vi "参数设置页.vi"() -> ()   [LabVIEW 2016, in "斯坦道氨氮V2.lvlib"]
uses:
  <vilib>/Plasmionique/MB Master/MB_Master/MB_Master.lvclass
  <vilib>/ptbypt/NI_PtbyPt.lvlib
panel:
  out "连接状态":bool
  out "低量程上限":dbl caption="低量程上限："
  out "数据刷新时间":string
  in  "通讯连接":bool=TRUE
  out "MB table":enum32{"Serial", "TCP"}(tab)
  in  "请选择串口:":refnum<visa-resource-name>
  in  "IP":string="127.0.0.1"
  in  "PORT":string="1001"
  in  "通信方式选择":enum16{"串口", "TCP"}(ring)
  in  "刷新":bool
  in  "测量模式":enum16{"跨度核查", "水样测量", "零点核查", "标样核查", "加标回收"}(ring)
  in  "参数下拉列表":u16(ring)
  in  "量程下拉列表":enum16{"低量程", "高量程"}(ring)
  in  "测试流程路径":path=path "data/流程.xml"
  in  "标样核查量程模式":T1 caption="标样核查："
  in  "加标回收量程模式":T1 caption="加标回收："
  in  "跨度核查量程模式":T1 caption="跨度核查："
  in  "零点核查量程模式":T1 caption="零点核查："
  in  "水样测试量程模式":T1 caption="水样测试："
  out "阈值（高->低）":dbl caption="阈值（高->低）："
  out "阈值（低->高）":dbl caption="阈值（低->高）："
  out "量程下限":dbl caption="量程下限："
  out "高量程上限":dbl caption="高量程上限："
  out "检出限":dbl caption="检出限："
  out "曲线截距":dbl caption="曲线截距：" format="%#.6f"
  out "曲线斜率":dbl caption="曲线斜率：" format="%#.6f"
  out "二次多项式系数":dbl caption="二次多项式系数：" format="%#.6f"
  out "消解时长":dbl caption="消解时长："
  out "消解温度":dbl caption="消解温度："
  out "测量精度":u16 caption="测量精度："
  in  "标样核查标液浓度":dbl caption="标样核查标液浓度："
  in  "跨度核查标液浓度":dbl caption="跨度核查标液浓度："
  in  "零点核查标液浓度":dbl caption="零点核查标液浓度："
  in  "跨度值":dbl caption="跨度值："
  # "自动量程设置"
  # "mg/L"
  # "mg/L"
  # "mg/L"
  # "mg/L"
  # "mg/L"
  # "mg/L"
  # "min"
  # "℃"
  # "mg/L"
  # "mg/L"
  # "mg/L"
  # "mg/L"
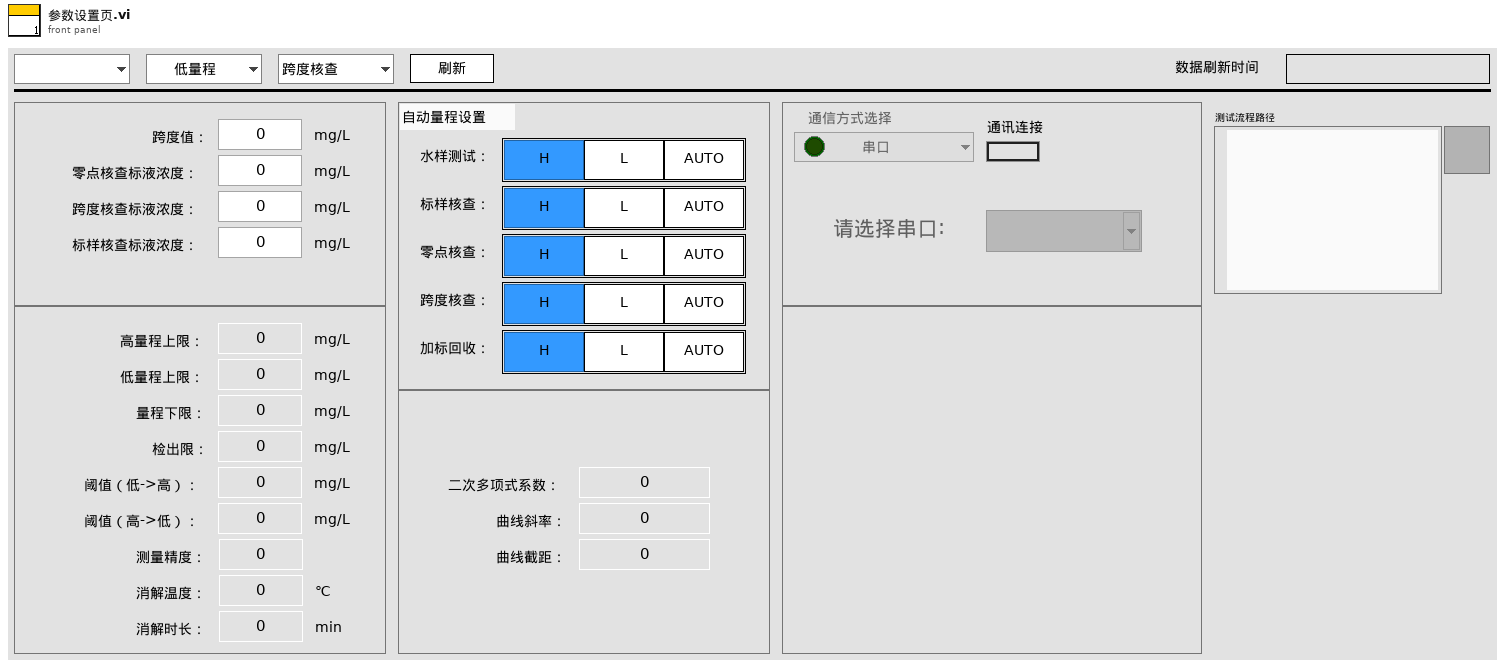
[diagram p1: front panel]
types:
  T1 = typedef "斯坦道氨氮V2.lvlib/量程设置.ctl" = enum32{"H", "L", "AUTO"}
  T2 = enum16{"跨度核查", "水样测量", "零点核查", "标样核查", "加标回收", "快捷测试", "空白校准", "标样校准"}
  T3 = typedef "LVStringsAndValuesArrayTypeDef_U16.ctl" = cluster{"String":string, "Value":u16}[]
  T4 = enum8{"Enabled", "Disabled", "Disabled and Grayed Out"}
  T5 = cluster{"总磷跨度值":dbl, "总磷零点标准液浓度":dbl, "总磷跨度标准液浓度":dbl, "总磷标准液标准浓度":dbl, "总氮跨度值":dbl, "总氮零点标准液浓度":dbl, "总氮跨度标准液浓度":dbl, "总氮标准液标准浓度":dbl, "氨氮跨度值":dbl, "氨氮零点标准液浓度":dbl, "氨氮跨度标准液浓度":dbl, "氨氮标准液标准浓度":dbl}
  T6 = cluster{"水样测试量程模式":enum16{"H", "L", "AUTO"}, "空白核查量程模式":enum16{"H", "L", "AUTO"}, "跨度核查量程模式":enum16{"H", "L", "AUTO"}, "加标回收量程模式":enum16{"H", "L", "AUTO"}, "标样核查量程模式":enum16{"H", "L", "AUTO"}}
  T7 = cluster{"水样测试量程模式":u16, "空白核查量程模式":u16, "跨度核查量程模式":u16, "加标回收量程模式":u16, "标样核查量程模式":u16}
  T8 = cluster{"精度":dbl, "检出限":dbl, "量程上限":dbl, "量程下限":dbl}
  T9 = cluster{"水样测试量程模式":T1, "零点核查量程模式":T1, "跨度核查量程模式":T1, "加标回收量程模式":T1, "标样核查量程模式":T1}
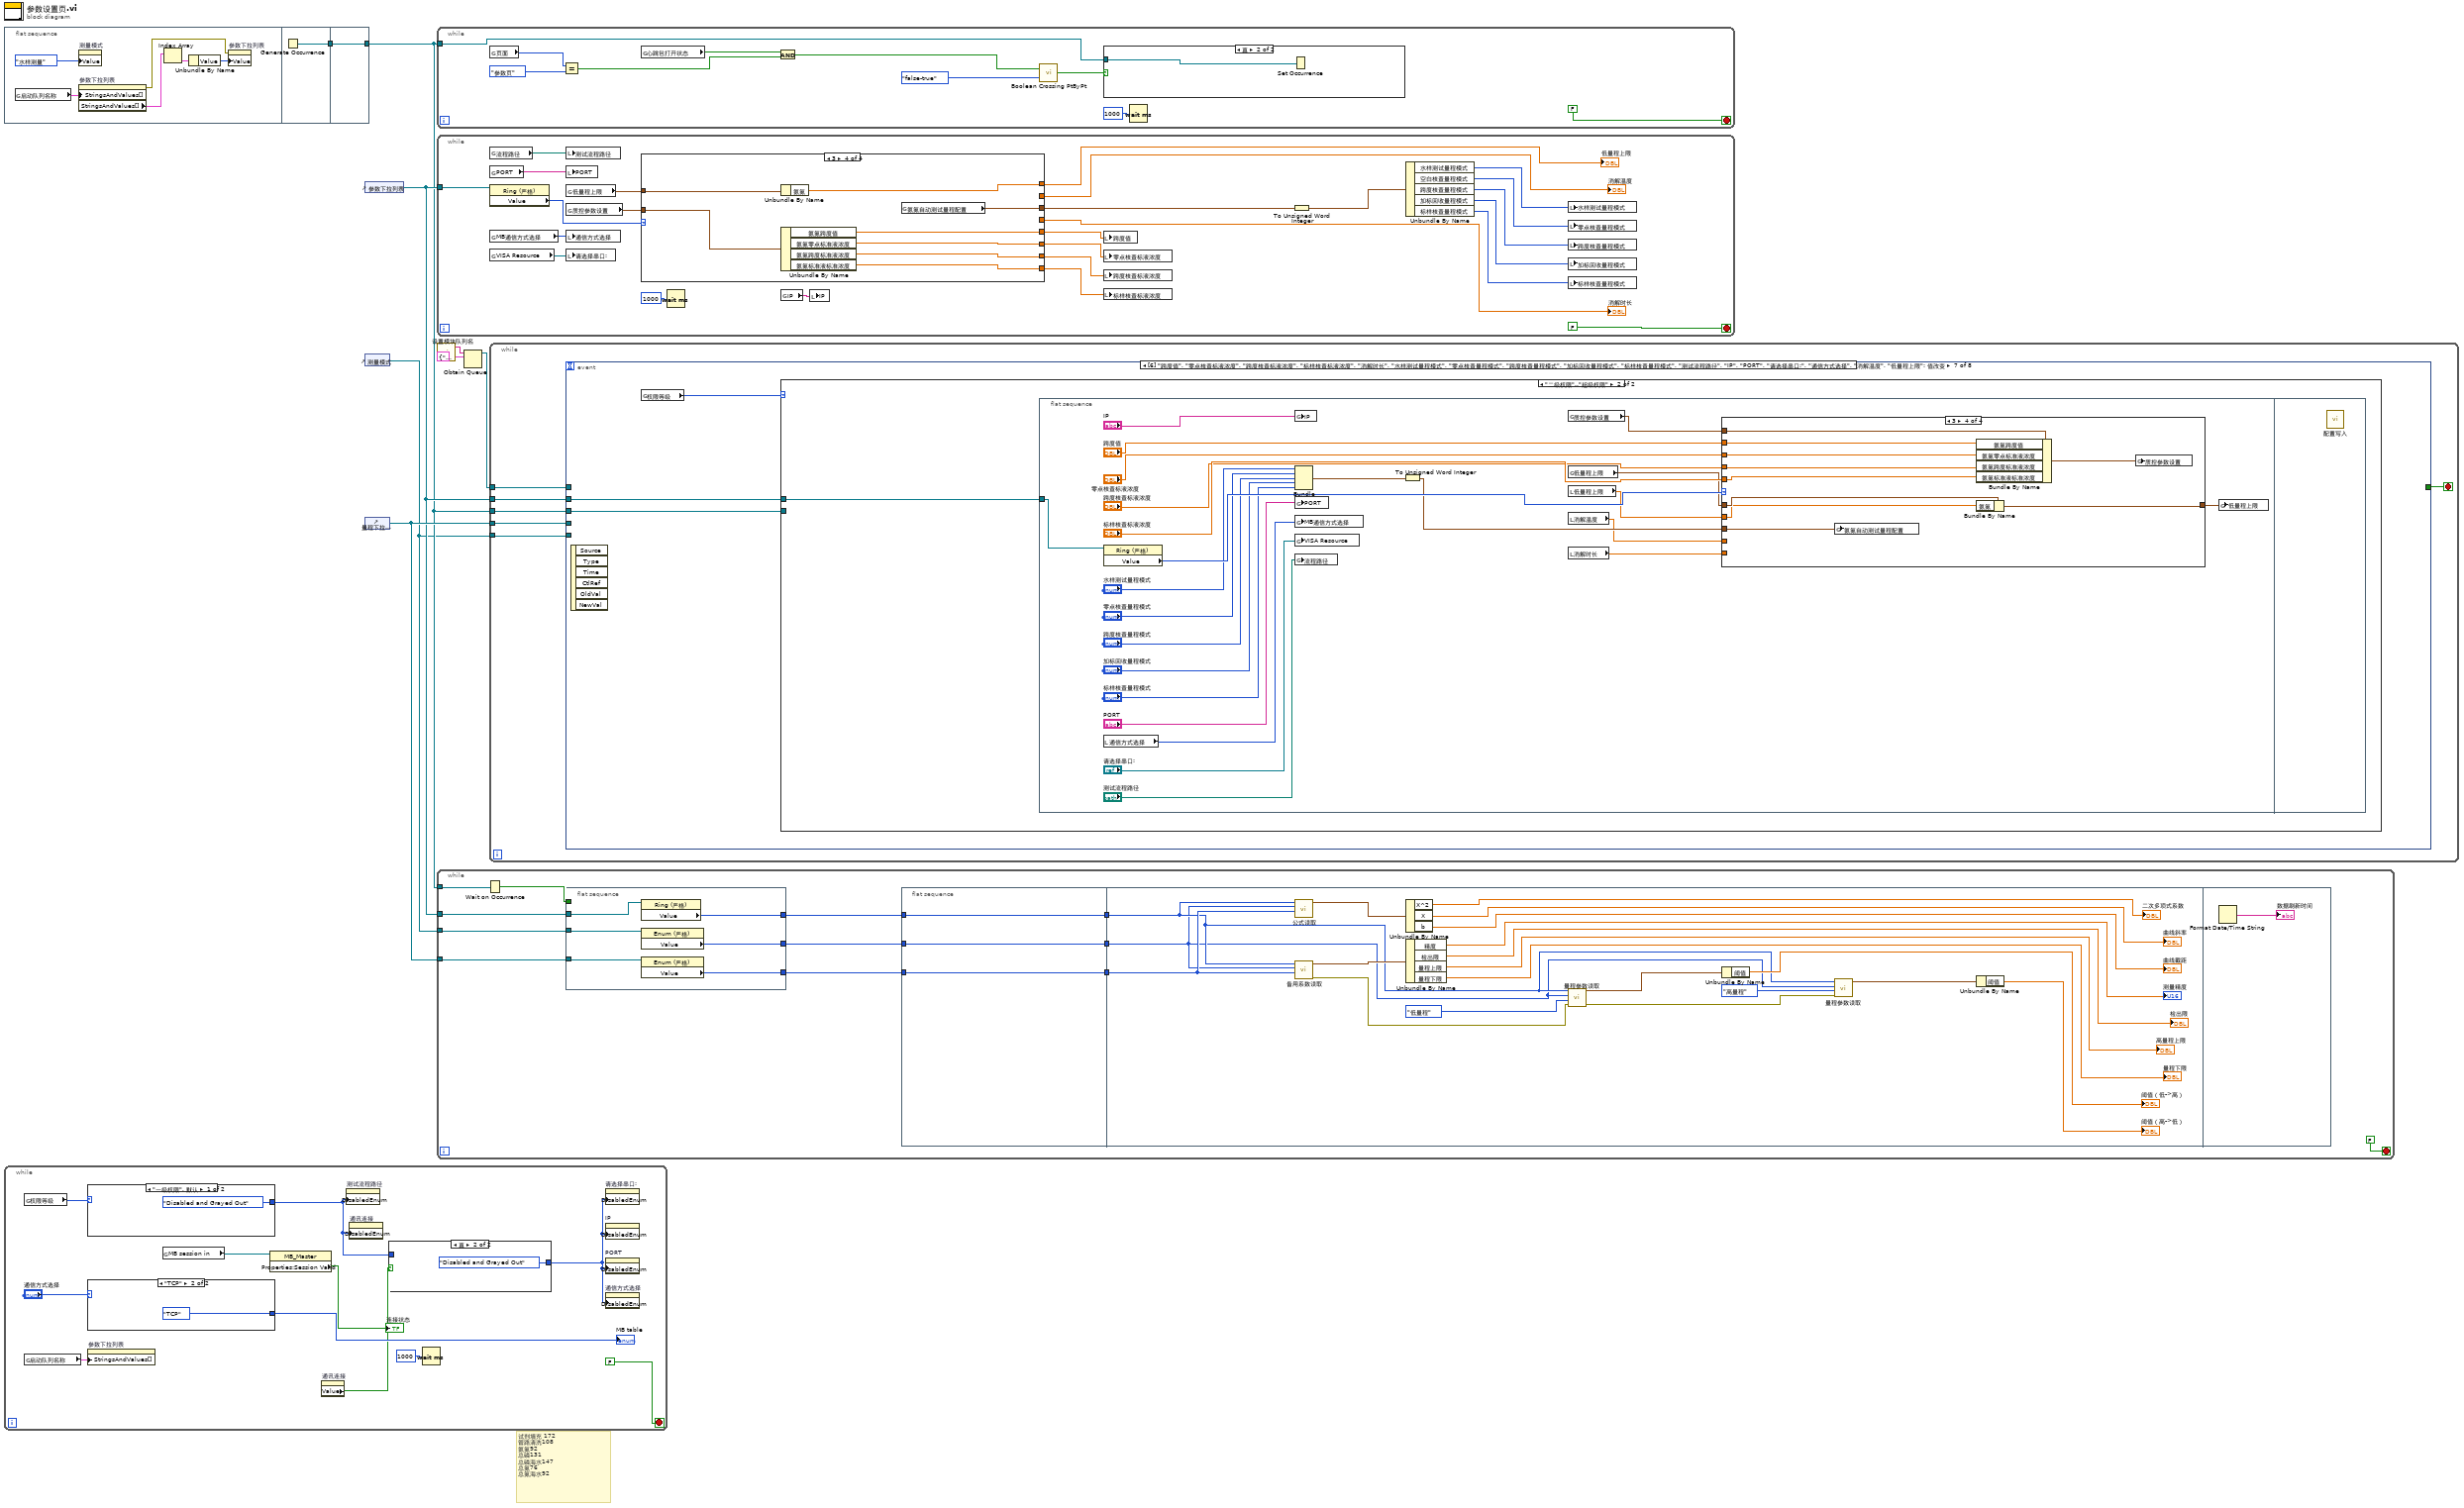
[diagram p0: block diagram]
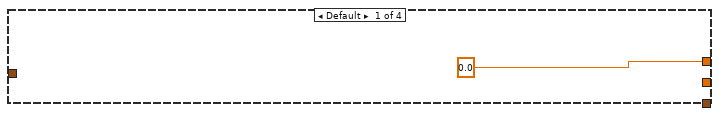
[diagram p3: hidden frame]
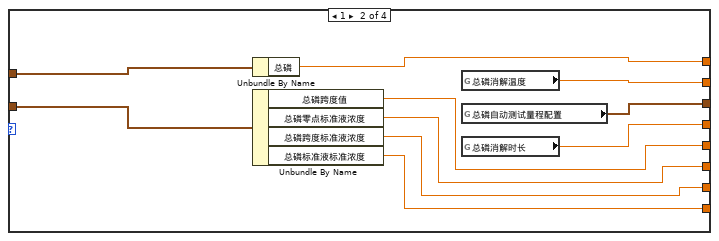
[diagram p4: hidden frame]
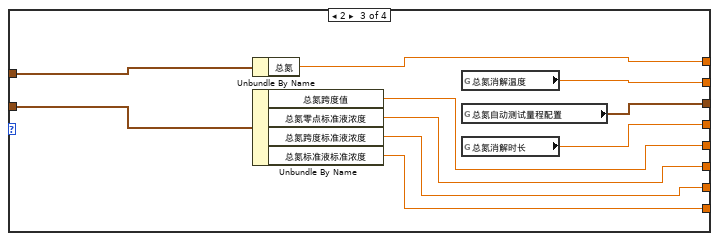
[diagram p5: hidden frame]
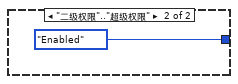
[diagram p6: hidden frame]
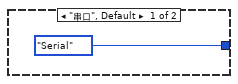
[diagram p7: hidden frame]
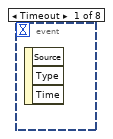
[diagram p9: hidden frame]
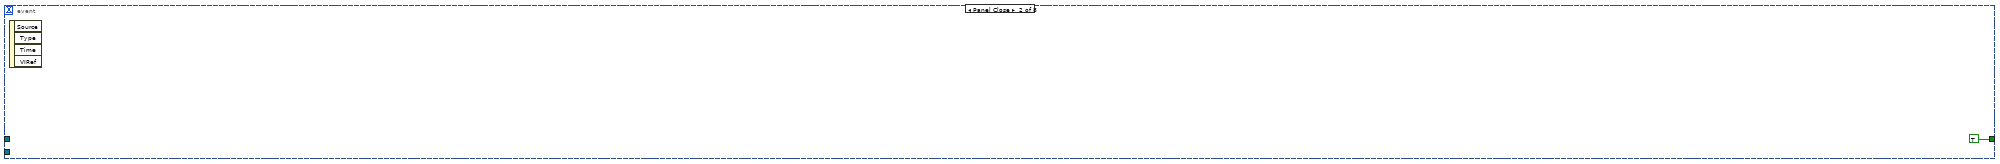
[diagram p10: hidden frame]
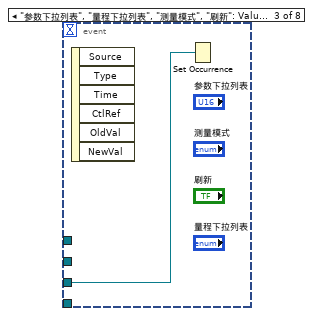
[diagram p11: hidden frame]
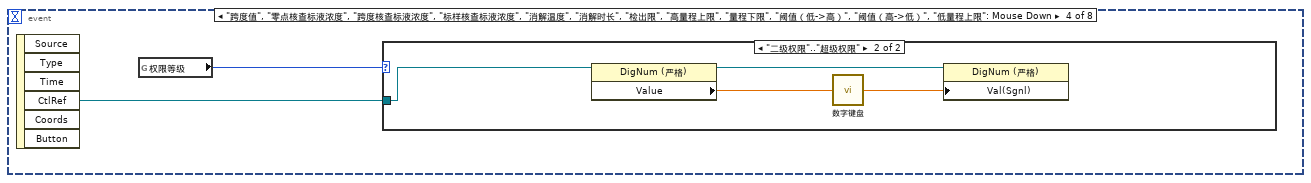
[diagram p12: hidden frame]
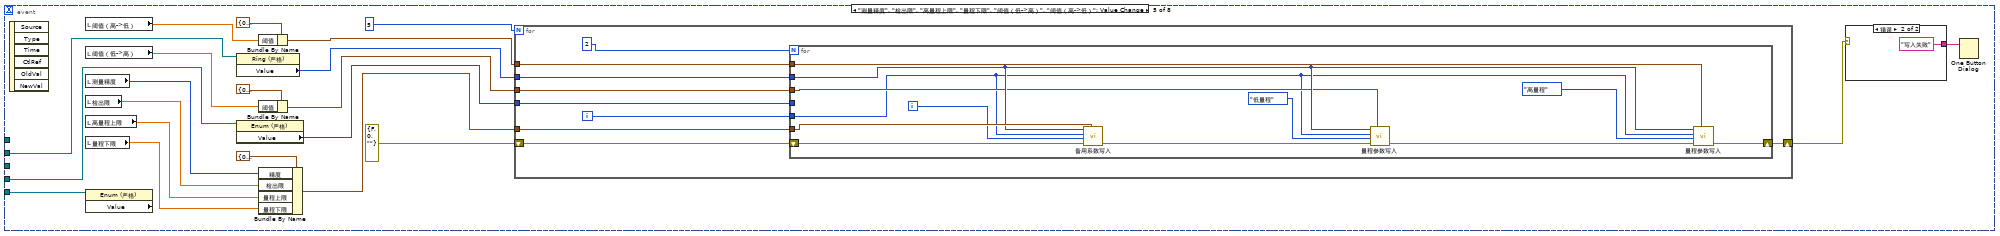
[diagram p14: hidden frame]
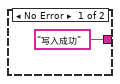
[diagram p15: hidden frame]
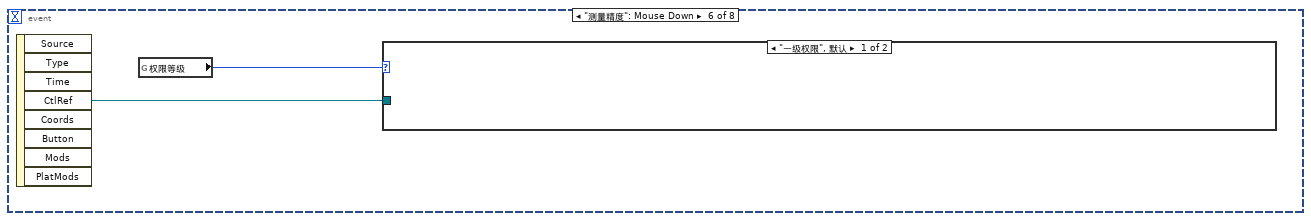
[diagram p16: hidden frame]
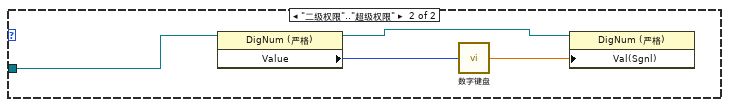
[diagram p17: hidden frame]
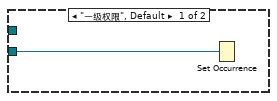
[diagram p18: hidden frame]
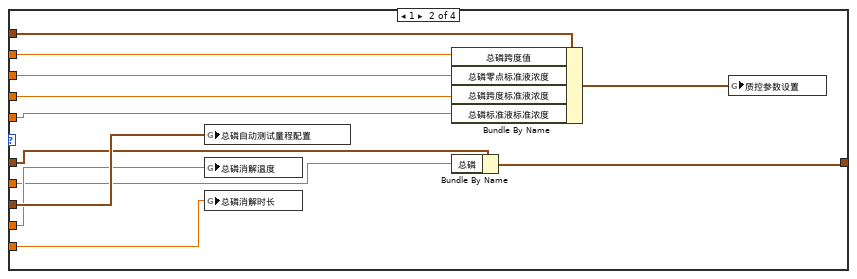
[diagram p20: hidden frame]
diagram:
  # "试剂填充 172 \n管路清洗108\n氨氮92\n总磷131\n总磷海水147\n总氮76\n总氮海水92"
  n1 = flat-sequence {
    tunnel: [w15] -> w8
    tunnel: [w16] -> w2
    tunnel: w8 -> [w16]
    frame #0 {
      n2 = global read "总磷总氮断电保存全局变量.vi" "启动队列名称"() -> (w10:cluster{"String":string, "Value":u16}[])
      n3 = property on="测量模式" class="Enum (严格)"("Value"=T2."水样测量" ("测量模式")) -> ()  [unwired: 2 in, 2 out]
      n4 = property on="参数下拉列表" class="Ring (严格)"("StringsAndValues[]"=w10) -> (error out=w13:errorcluster, "StringsAndValues[]"=w11:T3)  [unwired: 2 in, 1 out]
      n5 = Index Array(array=w11) -> (element=w12:cluster{"String":string, "Value":u16})  [unwired: 1 in]
      n6 = Unbundle By Name(w12) -> ("Value"=w14:u16)
      n7 = property on="参数下拉列表" class="Ring (严格)"(error in=w13, "Value"=w14) -> ()  [unwired: 1 in, 2 out]
    }
    frame #1 {
      n8 = Generate Occurrence() -> (w15:refnum<k4>)
    }
    frame #2 {
    }
  }
  n9 = while {
    stop <- FALSE stop-if-true
    n10 = global read "VAR总磷总氮全局变量.vi" "权限等级"() -> (w21:enum16{"一级权限", "二级权限", "三级权限", "超级权限"})
    n11 = global read "总磷总氮断电保存全局变量.vi" "启动队列名称"() -> (w19:cluster{"String":string, "Value":u16}[])
    n12 = case shown="\"一级权限\", 默认" w21 {
      tunnel: [T4."Disabled and Grayed Out" ("禁用") T4."Enabled" ("禁用")] -> w20
      frame "一级权限", Default {
      }
      frame "二级权限".."超级权限" {
      }
    }
    n13 = case shown="\"TCP\"" "通信方式选择" {
      tunnel: [enum32{"Serial", "TCP"}."Serial" ("MB table") enum32{"Serial", "TCP"}."TCP" ("MB table")] -> w23
      frame "串口", Default {
      }
      frame "TCP" {
      }
    }
    "MB table" <- w23
    n14 = property on="参数下拉列表" class="Ring (严格)"("StringsAndValues[]"=w19) -> ()  [unwired: 2 in, 2 out]
    n15 = global read "VAR总磷总氮全局变量.vi" "MB session in"() -> (w26:refnum<class "MB_Master.lvclass">)
    n16 = property class="MB_Master"(reference=w26) -> ("Properties:Session Valid"=→"连接状态":bool)  [unwired: 1 in, 2 out]
    n17 = property on="通讯连接" class="Bool (严格)"() -> ("Value"=w17:bool)  [unwired: 2 in, 2 out]
    n18 = property on="测试流程路径" class="Path"("DisabledEnum"=w20) -> ()  [unwired: 2 in, 2 out]
    n19 = property on="通讯连接" class="Bool (严格)"("DisabledEnum"=w20) -> ()  [unwired: 2 in, 2 out]
    n20 = case shown="真" w17 {
      tunnel: [w32 T4."Disabled and Grayed Out" ("禁用")] -> w24
      tunnel: w20 -> [w32 _]
      frame False {
      }
      frame True {
      }
    }
    n21 = Wait (ms)(milliseconds to wait=u32 1000 ("等待时间（毫秒）")) -> ()  [unwired: 1 out]
    n22 = property on="请选择串口:" class="VISAName"("DisabledEnum"=w24) -> ()  [unwired: 2 in, 2 out]
    n23 = property on="IP" class="Str"("DisabledEnum"=w24) -> ()  [unwired: 2 in, 2 out]
    n24 = property on="PORT" class="Str"("DisabledEnum"=w24) -> ()  [unwired: 2 in, 2 out]
    n25 = property on="通信方式选择" class="Enum (严格)"("DisabledEnum"=w24) -> ()  [unwired: 2 in, 2 out]
  }
  n26 = control-ref of="参数下拉列表"() -> (w3:refnum<vi>)
  n27 = control-ref of="测量模式"() -> (w1:refnum<vi>)
  n28 = control-ref of="量程下拉列表"() -> (w4:refnum<vi>)
  n29 = while {
    tunnel: w2 -> [w40]
    stop <- FALSE stop-if-true
    n30 = global read "VAR总磷总氮全局变量.vi" "页面"() -> (w42:enum16{"主页", "参数页", "校准页"})
    n31 = Equal?(x=w42, y=enum16{"主页", "参数页", "校准页"}."参数页" ("页面")) -> (x = y?=w41:bool)
    n32 = global read "VAR总磷总氮全局变量.vi" "心跳包打开状态"() -> (w36:bool)
    n33 = And(x=w36, y=w41) -> (x .and. y?=w37:bool)
    n34 = call <vilib>:"Boolean Crossing PtByPt.vi"("direction"=enum16{"either", "false-true", "true-false"}."false-true", "input"=w37) -> ("crossing"=w35:bool)  [unwired: 1 in]
    n35 = case shown="真" w35 {
      tunnel: w40 -> [_ w44]
      frame False {
      }
      frame True {
        n36 = Set Occurrence(w44) -> ()
      }
    }
    n37 = Wait (ms)(milliseconds to wait=u32 1000 ("等待时间（毫秒）")) -> ()  [unwired: 1 out]
  }
  n38 = while {
    tunnel: w3 -> [w49]
    stop <- FALSE stop-if-true
    n39 = global read "总磷总氮断电保存全局变量.vi" "流程路径"() -> (w64:path)
    n40 = global read "总磷总氮断电保存全局变量.vi" "PORT"() -> (w66:string)
    n41 = property class="Ring (严格)"(reference=w49) -> ("Value"=w48:u16)  [unwired: 1 in, 2 out]
    n42 = global read "总磷总氮断电保存全局变量.vi" "MB通信方式选择"() -> (w63:enum16{"串口", "TCP"})
    n43 = global read "总磷总氮断电保存全局变量.vi" "VISA Resource"() -> (w67:refnum<visa-resource-name>)
    n44 = local write "测试流程路径"(w64) -> ()
    n45 = local write "PORT"(w66) -> ()
    n46 = global read "总磷总氮断电保存全局变量.vi" "低量程上限"() -> (w46:cluster{"总磷":dbl, "总氮":dbl, "氨氮":dbl})
    n47 = global read "总磷总氮断电保存全局变量.vi" "质控参数设置"() -> (w58:T5)
    n48 = local write "通信方式选择"(w63) -> ()
    n49 = local write "请选择串口:"(w67) -> ()
    n50 = case shown="3" w48 {
      tunnel: [_ w80 w90 w98] -> w56
      tunnel: [_ w79 w89 _] -> w57
      tunnel: w58 -> [_ w78 w88 w97]
      tunnel: [_ w77 w87 w96] -> w59
      tunnel: [_ w76 w86 w95] -> w60
      tunnel: [_ w75 w85 w94] -> w61
      tunnel: [_ w74 w84 w93] -> w62
      tunnel: [_ w73 w83 _] -> w47
      tunnel: w46 -> [_ w72 w82 w92]
      tunnel: [0.0 ("COD") w71 w81 w91] -> w45
      frame Default {
      }
      frame 1 {
        n51 = Unbundle By Name(w72) -> ("总磷"=w71:dbl)
        n52 = Unbundle By Name(w78) -> ("总磷跨度值"=w77:dbl, "总磷零点标准液浓度"=w76:dbl, "总磷跨度标准液浓度"=w75:dbl, "总磷标准液标准浓度"=w74:dbl)
        n53 = global read "总磷总氮断电保存全局变量.vi" "总磷消解温度"() -> (w73:dbl)
        n54 = global read "总磷总氮断电保存全局变量.vi" "总磷自动测试量程配置"() -> (w80:T6)
        n55 = global read "总磷总氮断电保存全局变量.vi" "总磷消解时长"() -> (w79:dbl)
      }
      frame 2 {
        n56 = Unbundle By Name(w82) -> ("总氮"=w81:dbl)
        n57 = Unbundle By Name(w88) -> ("总氮跨度值"=w87:dbl, "总氮零点标准液浓度"=w86:dbl, "总氮跨度标准液浓度"=w85:dbl, "总氮标准液标准浓度"=w84:dbl)
        n58 = global read "总磷总氮断电保存全局变量.vi" "总氮消解温度"() -> (w83:dbl)
        n59 = global read "总磷总氮断电保存全局变量.vi" "总氮自动测试量程配置"() -> (w90:T6)
        n60 = global read "总磷总氮断电保存全局变量.vi" "总氮消解时长"() -> (w89:dbl)
      }
      frame 3 {
        n61 = Unbundle By Name(w92) -> ("氨氮"=w91:dbl)
        n62 = Unbundle By Name(w97) -> ("氨氮跨度值"=w96:dbl, "氨氮零点标准液浓度"=w95:dbl, "氨氮跨度标准液浓度"=w94:dbl, "氨氮标准液标准浓度"=w93:dbl)
        n63 = global read "总磷总氮断电保存全局变量.vi" "氨氮自动测试量程配置"() -> (w98:T6)
      }
    }
    "消解时长" <- w57
    "消解温度" <- w47
    "低量程上限" <- w45
    n64 = Wait (ms)(milliseconds to wait=u32 1000 ("等待时间（毫秒）")) -> ()  [unwired: 1 out]
    n65 = global read "总磷总氮断电保存全局变量.vi" "IP"() -> (w65:string)
    n66 = local write "IP"(w65) -> ()
    n67 = local write "跨度值"(w59) -> ()
    n68 = local write "零点核查标液浓度"(w60) -> ()
    n69 = local write "跨度核查标液浓度"(w61) -> ()
    n70 = local write "标样核查标液浓度"(w62) -> ()
    n71 = To Unsigned Word Integer(number=w56) -> (unsigned 16bit integer=w55:T7)
    n72 = Unbundle By Name(w55) -> ("水样测试量程模式"=w54:u16, "空白核查量程模式"=w52:u16, "跨度核查量程模式"=w51:u16, "加标回收量程模式"=w50:u16, "标样核查量程模式"=w53:u16)
    n73 = local write "水样测试量程模式"(w54) -> ()
    n74 = local write "零点核查量程模式"(w52) -> ()
    n75 = local write "跨度核查量程模式"(w51) -> ()
    n76 = local write "加标回收量程模式"(w50) -> ()
    n77 = local write "标样核查量程模式"(w53) -> ()
  }
  n78 = call "设置模块队列名.vi"() -> ("Msg"=w6:string)  [unwired: 5 in]
  n79 = while {
    tunnel: w3 -> [w109]
    tunnel: w4 -> [w108]
    tunnel: w1 -> [w107]
    tunnel: w2 -> [w106]
    stop <- FALSE stop-if-true
    n80 = Wait on Occurrence(2:w106) -> (0:w100:bool)  [unwired: 2 in]
    n81 = flat-sequence {
      tunnel: w109 -> [w116]
      tunnel: w108 -> [w115]
      tunnel: w107 -> [w114]
      tunnel: [w113] -> w103
      tunnel: [w112] -> w102
      tunnel: [w111] -> w101
      tunnel: w100 -> [_]
      frame #0 {
        n82 = property class="Ring (严格)"(reference=w116) -> ("Value"=w113:u16)  [unwired: 1 in, 2 out]
        n83 = property class="Enum (严格)"(reference=w114) -> ("Value"=w111:enum16{"跨度核查", "水样测量", "零点核查", "标样核查", "加标回收"})  [unwired: 1 in, 2 out]
        n84 = property class="Enum (严格)"(reference=w115) -> ("Value"=w112:enum16{"低量程", "高量程"})  [unwired: 1 in, 2 out]
      }
    }
    n85 = flat-sequence {
      tunnel: [w119] -> w105
      tunnel: [w118] -> w104
      tunnel: w103 -> [w117]
      tunnel: w102 -> [w119]
      tunnel: w101 -> [w118]
      tunnel: [w117] -> w99
      tunnel: w105 -> [w134]
      tunnel: w104 -> [w124]
      tunnel: w99 -> [w125]
      frame #0 {
      }
      frame #1 {
        n86 = call "公式读取.vi"("量程下拉列表"=w134, "测量模式"=w124, "参数下拉列表"=w125) -> ("公式"=w139:cluster{"X^2":dbl, "X":dbl, "b":dbl})  [unwired: 7 in, 1 out]
        n87 = call "备用系数读取.vi"("量程下拉列表"=w134, "测量模式"=w124, "参数下拉列表"=w125) -> ("error out"=w135:errorcluster, "备用系数"=w133:T8)  [unwired: 7 in]
        n88 = Unbundle By Name(w139) -> ("X^2"=→"二次多项式系数":dbl, "X"=→"曲线斜率":dbl, "b"=→"曲线截距":dbl)
        n89 = Unbundle By Name(w133) -> ("精度"=→"测量精度":dbl, "检出限"=→"检出限":dbl, "量程上限"=→"高量程上限":dbl, "量程下限"=→"量程下限":dbl)
        n90 = call "量程参数读取.vi"("error in (no error)"=w135, "量程下拉列表"=enum16{"低量程", "高量程"}."低量程", "测量模式"=w124, "参数下拉列表"=w125) -> ("error out"=w126:errorcluster, "量程切换阈值"=w132:cluster{"阈值":dbl, "标液浓度":dbl})  [unwired: 6 in]
        n91 = Unbundle By Name(w132) -> ("阈值"=→"阈值（低->高）":dbl)
        n92 = call "量程参数读取.vi"("error in (no error)"=w126, "量程下拉列表"=enum16{"低量程", "高量程"}."高量程", "测量模式"=w124, "参数下拉列表"=w125) -> ("量程切换阈值"=w121:cluster{"阈值":dbl, "标液浓度":dbl})  [unwired: 6 in, 1 out]
        n93 = Unbundle By Name(w121) -> ("阈值"=→"阈值（高->低）":dbl)
      }
      frame #2 {
        n94 = Format Date/Time String() -> (date/time string=→"数据刷新时间":string)  [unwired: 3 in]
      }
    }
  }
  n95 = Obtain Queue(name (unnamed)=w6, element data type=cluster{"命令":string, "data":variant} {"命令"="", "data"=variant}) -> (queue out=w5:refnum<queue>)  [unwired: 3 in, 2 out]
  n96 = while {
    tunnel: w2 -> [w145]
    tunnel: w3 -> [w144]
    tunnel: w5 -> [w143]
    tunnel: w4 -> [w142]
    tunnel: w1 -> [w141]
    stop <- w146 stop-if-true
    n97 = event shown="[6] \"跨度值\", \"零点核查标液浓度\", \"跨度核查标液浓度\", \"标样核查标液浓度\", \"消解时长\", \"水样测试量程模式\", \"零点核查量程模式\", \"跨度核查量程模式\", \"加标回收量程模式\", \"标样核查量程模式\", \"测试流程路径\", \"IP\", \"PORT\", \"请选择串口:\", \"通信方式选择\", \"消解温度\", \"低量程上限\": 值改变" {
      selector: _ -> [_ _ _ _ _ _ _ _]
      dyn-events: _ -> [_ _ _ _ _ _ _ _]
      timeout: _ -> [_ _ _ _ _ _ _ _]
      tunnel: [_ TRUE _ _ _ _ _ _] -> w146
      tunnel: w145 -> [_ _ w148 _ _ _ w205 _]
      tunnel: w144 -> [_ _ _ _ w175 _ w207 _]
      tunnel: w143 -> [_ _ _ _ _ _ _ w270]
      tunnel: w142 -> [_ _ _ _ w168 _ _ _]
      tunnel: w141 -> [_ _ _ _ w169 _ _ _]
      event Timeout {
        n98 = event-data() -> ()  [unwired: 1 in, 3 out]
      }
      event Panel Close {
        n99 = event-data() -> ()  [unwired: 1 in, 4 out]
      }
      event "参数下拉列表", "量程下拉列表", "测量模式", "刷新": Value Change {
        n100 = event-data() -> ()  [unwired: 1 in, 6 out]
        n101 = Set Occurrence(w148) -> ()
      }
      event "跨度值", "零点核查标液浓度", "跨度核查标液浓度", "标样核查标液浓度", "消解温度", "消解时长", "检出限", "高量程上限", "量程下限", "阈值（低->高）", "阈值（高->低）", "低量程上限": Mouse Down {
        n102 = event-data() -> ("CtlRef"=w150:refnum<vi>)  [unwired: 1 in, 5 out]
        n103 = global read "VAR总磷总氮全局变量.vi" "权限等级"() -> (w149:enum16{"一级权限", "二级权限", "三级权限", "超级权限"})
        n104 = case shown="\"二级权限\"..\"超级权限\"" w149 {
          tunnel: w150 -> [_ w154]
          frame "一级权限", Default {
          }
          frame "二级权限".."超级权限" {
            n105 = property class="DigNum (严格)"(reference=w154) -> (reference out=w152:refnum<vi>, "Value"=w153:dbl)  [unwired: 1 in, 1 out]
            n106 = call "数字键盘.vi"("OldNumber"=w153) -> ("NewNumber"=w151:dbl)
            n107 = property class="DigNum (严格)"(reference=w152, "Val(Sgnl)"=w151) -> ()  [unwired: 1 in, 2 out]
          }
        }
      }
      event "测量精度", "检出限", "高量程上限", "量程下限", "阈值（低->高）", "阈值（高->低）": Value Change {
        n108 = event-data() -> ()  [unwired: 1 in, 6 out]
        n109 = local read "阈值（高->低）"() -> (w158:dbl)
        n110 = local read "阈值（低->高）"() -> (w163:dbl)
        n111 = local read "测量精度"() -> (w171:u16)
        n112 = local read "检出限"() -> (w172:dbl)
        n113 = local read "高量程上限"() -> (w174:dbl)
        n114 = local read "量程下限"() -> (w173:dbl)
        n115 = property class="Enum (严格)" props=["Value"](reference=w169) -> ()  [unwired: 1 in, 3 out]
        n116 = property class="Ring (严格)"(reference=w175) -> ("Value"=w162:u16)  [unwired: 1 in, 2 out]
        n117 = property class="Enum (严格)"(reference=w168) -> ("Value"=w167:enum16{"低量程", "高量程"})  [unwired: 1 in, 2 out]
        n118 = Bundle By Name(cluster=cluster{"阈值":dbl, "标液浓度":dbl} {"阈值"=0.0, "标液浓度"=0.0} ("量程切换阈值"), "阈值"=w158) -> (w159:cluster{"阈值":dbl, "标液浓度":dbl})
        n119 = Bundle By Name(cluster=cluster{"阈值":dbl, "标液浓度":dbl} {"阈值"=0.0, "标液浓度"=0.0} ("量程切换阈值"), "阈值"=w163) -> (w161:cluster{"阈值":dbl, "标液浓度":dbl})
        n120 = Bundle By Name(cluster=T8 {"精度"=0.0, "检出限"=0.0, "量程上限"=0.0, "量程下限"=0.0} ("备用系数"), "精度"=w171, "检出限"=w172, "量程上限"=w174, "量程下限"=w173) -> (w165:T8)
        n121 = for {
          N: 5 -> [_]
          tunnel: w167 -> [w184]
          tunnel: w165 -> [w183]
          tunnel: w162 -> [w182]
          tunnel: w161 -> [w181]
          tunnel: w159 -> [w180]
          shift-right: [w179] -> w157
          shift-left: errorcluster {"status"=FALSE, "code"=0, "source"=""} ("error out") -> [w176]
          i -> [w177]
          n122 = for {
            N: 2 -> [_]
            tunnel: w184 -> [_]
            tunnel: w183 -> [w196]
            tunnel: w182 -> [w192]
            tunnel: w181 -> [w190]
            tunnel: w180 -> [w189]
            tunnel: w177 -> [w186]
            shift-right: [w188] -> w179
            shift-left: w176 -> [w185]
            i -> [w187]
            n123 = call "备用系数写入.vi"("备用系数"=w196, "error in (no error)"=w185, "量程下拉列表"=w187, "测量模式"=w186, "参数下拉列表"=w192) -> ("error out"=w195:errorcluster)  [unwired: 6 in]
            n124 = call "量程参数写入.vi"("量程切换阈值"=w190, "error in (no error)"=w195, "量程下拉列表"=enum16{"低量程", "高量程"}."低量程", "测量模式"=w186, "参数下拉列表"=w192) -> ("error out"=w193:errorcluster)  [unwired: 6 in]
            n125 = call "量程参数写入.vi"("量程切换阈值"=w189, "error in (no error)"=w193, "量程下拉列表"=enum16{"低量程", "高量程"}."高量程", "测量模式"=w186, "参数下拉列表"=w192) -> ("error out"=w188:errorcluster)  [unwired: 6 in]
          }
        }
        n126 = case shown="错误" w157 {
          tunnel: ["写入成功" "写入失败"] -> w170
          frame No Error {
          }
          frame Error {
          }
        }
        n127 = One Button Dialog(message=w170) -> ()  [unwired: 1 in, 1 out]
      }
      event "测量精度": Mouse Down {
        n128 = event-data() -> ("CtlRef"=w200:refnum<vi>)  [unwired: 1 in, 7 out]
        n129 = global read "VAR总磷总氮全局变量.vi" "权限等级"() -> (w199:enum16{"一级权限", "二级权限", "三级权限", "超级权限"})
        n130 = case shown="\"一级权限\", 默认" w199 {
          tunnel: w200 -> [_ w204]
          frame "一级权限", Default {
          }
          frame "二级权限".."超级权限" {
            n131 = property class="DigNum (严格)"(reference=w204) -> (reference out=w202:refnum<vi>, "Value"=w203:u16)  [unwired: 1 in, 1 out]
            n132 = call "数字键盘.vi"("OldNumber"=w203) -> ("NewNumber"=w201:dbl)
            n133 = property class="DigNum (严格)"(reference=w202, "Val(Sgnl)"=w201) -> ()  [unwired: 1 in, 2 out]
          }
        }
      }
      event "跨度值", "零点核查标液浓度", "跨度核查标液浓度", "标样核查标液浓度", "消解时长", "测试流程路径", "IP", "PORT", "请选择串口:", "通信方式选择", "消解温度", "低量程上限": Value Change {
        n134 = event-data() -> ()  [unwired: 1 in, 6 out]
        n135 = global read "VAR总磷总氮全局变量.vi" "权限等级"() -> (w206:enum16{"一级权限", "二级权限", "三级权限", "超级权限"})
        n136 = case shown="\"二级权限\"..\"超级权限\"" w206 {
          tunnel: w207 -> [_ w209]
          tunnel: w205 -> [w208 _]
          frame "一级权限", Default {
            n137 = Set Occurrence(w208) -> ()
          }
          frame "二级权限".."超级权限" {
            n138 = flat-sequence {
              tunnel: w209 -> [w232]
              frame #0 {
                n139 = property class="Ring (严格)"(reference=w232) -> ("Value"=w231:u16)  [unwired: 1 in, 2 out]
                n140 = local read "通信方式选择"() -> (w215:enum16{"串口", "TCP"})
                n141 = global write "总磷总氮断电保存全局变量.vi" "IP"("IP") -> ()
                n142 = Bundle("水样测试量程模式"="水样测试量程模式", "零点核查量程模式"="零点核查量程模式", "跨度核查量程模式"="跨度核查量程模式", "加标回收量程模式"="加标回收量程模式", "标样核查量程模式"="标样核查量程模式") -> (w220:T9)  [unwired: 1 in]
                n143 = global write "总磷总氮断电保存全局变量.vi" "PORT"("PORT") -> ()
                n144 = global write "总磷总氮断电保存全局变量.vi" "MB通信方式选择"(w215) -> ()
                n145 = global write "总磷总氮断电保存全局变量.vi" "VISA Resource"("请选择串口:") -> ()
                n146 = global write "总磷总氮断电保存全局变量.vi" "流程路径"("测试流程路径") -> ()
                n147 = To Unsigned Word Integer(number=w220) -> (unsigned 16bit integer=w219:cluster{u16, u16, u16, u16, u16})
                n148 = global read "总磷总氮断电保存全局变量.vi" "质控参数设置"() -> (w226:T5)
                n149 = global read "总磷总氮断电保存全局变量.vi" "低量程上限"() -> (w212:cluster{"总磷":dbl, "总氮":dbl, "氨氮":dbl})
                n150 = local read "低量程上限"() -> (w210:dbl)
                n151 = local read "消解温度"() -> (w213:dbl)
                n152 = local read "消解时长"() -> (w214:dbl)
                n153 = case shown="3" w231 {
                  tunnel: "跨度值" -> [_ w244 w256 w266]
                  tunnel: "标样核查标液浓度" -> [_ w241 w253 w263]
                  tunnel: "跨度核查标液浓度" -> [_ w242 w254 w264]
                  tunnel: "零点核查标液浓度" -> [_ w243 w255 w265]
                  tunnel: w226 -> [_ w246 w258 w268]
                  tunnel: w219 -> [_ w240 w252 w262]
                  tunnel: w214 -> [_ w239 w251 _]
                  tunnel: w213 -> [_ w238 w250 _]
                  tunnel: w212 -> [w234 w237 w249 w261]
                  tunnel: [w234 w236 w248 w260] -> w211
                  tunnel: w210 -> [_ w235 w247 w259]
                  frame 0, Default {
                  }
                  frame 1 {
                    n154 = global write "总磷总氮断电保存全局变量.vi" "总磷自动测试量程配置"(w240) -> ()
                    n155 = global write "总磷总氮断电保存全局变量.vi" "总磷消解温度"(w238) -> ()
                    n156 = global write "总磷总氮断电保存全局变量.vi" "总磷消解时长"(w239) -> ()
                    n157 = Bundle By Name(cluster=w246, "总磷跨度值"=w244, "总磷零点标准液浓度"=w243, "总磷跨度标准液浓度"=w242, "总磷标准液标准浓度"=w241) -> (w245:T5)
                    n158 = Bundle By Name(cluster=w237, "总磷"=w235) -> (w236:cluster{"总磷":dbl, "总氮":dbl, "氨氮":dbl})
                    n159 = global write "总磷总氮断电保存全局变量.vi" "质控参数设置"(w245) -> ()
                  }
                  frame 2 {
                    n160 = global write "总磷总氮断电保存全局变量.vi" "总氮自动测试量程配置"(w252) -> ()
                    n161 = global write "总磷总氮断电保存全局变量.vi" "总氮消解温度"(w250) -> ()
                    n162 = global write "总磷总氮断电保存全局变量.vi" "总氮消解时长"(w251) -> ()
                    n163 = Bundle By Name(cluster=w258, "总氮跨度值"=w256, "总氮零点标准液浓度"=w255, "总氮跨度标准液浓度"=w254, "总氮标准液标准浓度"=w253) -> (w257:T5)
                    n164 = Bundle By Name(cluster=w249, "总氮"=w247) -> (w248:cluster{"总磷":dbl, "总氮":dbl, "氨氮":dbl})
                    n165 = global write "总磷总氮断电保存全局变量.vi" "质控参数设置"(w257) -> ()
                  }
                  frame 3 {
                    n166 = global write "总磷总氮断电保存全局变量.vi" "氨氮自动测试量程配置"(w262) -> ()
                    n167 = Bundle By Name(cluster=w268, "氨氮跨度值"=w266, "氨氮零点标准液浓度"=w265, "氨氮跨度标准液浓度"=w264, "氨氮标准液标准浓度"=w263) -> (w267:T5)
                    n168 = Bundle By Name(cluster=w261, "氨氮"=w259) -> (w260:cluster{"总磷":dbl, "总氮":dbl, "氨氮":dbl})
                    n169 = global write "总磷总氮断电保存全局变量.vi" "质控参数设置"(w267) -> ()
                  }
                }
                n170 = global write "总磷总氮断电保存全局变量.vi" "低量程上限"(w211) -> ()
              }
              frame #1 {
                n171 = call "配置写入.vi"() -> ()  [unwired: 11 in, 1 out]
              }
            }
          }
        }
      }
      event "通讯连接": Value Change {
        n172 = event-data() -> ("NewVal"=w269:bool)  [unwired: 1 in, 5 out]
        n173 = Flush Queue(queue=w270) -> (queue out=w271:refnum<queue>)  [unwired: 1 in, 2 out]
        n174 = case shown="假" w269 {
          tunnel: w271 -> [w272 w274]
          frame False {
            n175 = Enqueue Element(queue=w272, element=cluster{"命令":string, "data":variant} {"命令"="停用模块", "data"=variant} ("元素")) -> ()  [unwired: 2 in, 3 out]
          }
          frame True {
            n176 = Enqueue Element(queue=w274, element=cluster{"命令":string, "data":variant} {"命令"="启用模块", "data"=variant} ("元素")) -> ()  [unwired: 2 in, 3 out]
          }
        }
      }
    }
  }
